vi "LVPortProcessMatlabPropertyEvents.vi"(8 "error in":errorcluster, 10 "Wait for events [ms] (0)":i32, 11 "pID":string) -> (0 "error out":errorcluster)   [LabVIEW 2017]
uses:
  Properties/LVPortControlBindingInfoType.ctl
  Properties/LVPortControlBindingDirectionEnum.ctl
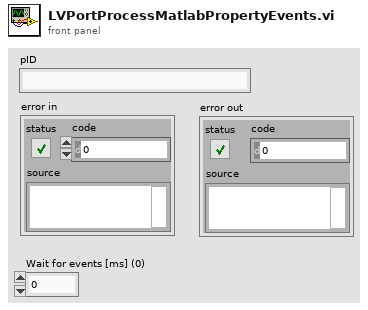
[diagram p1: front panel]
types:
  T1 = typedef "LVPortEventRegistrationDataType.ctl" = refnum<event-registration>
  T2 = typedef "LVPortControlBindingDirectionEnum.ctl" = enum16{"BiDirectional", "ToMatlab", "ToLabview"}
  T3 = typedef "LVPortControlBindingInfoType.ctl" = cluster{"Bound Control":refnum<vi>, "Name":string, "Direction":T2, "Event Register":refnum<event-registration>}
  T4 = typedef "Dictionary Object RefNum__ogtk.ctl" = refnum<k1>
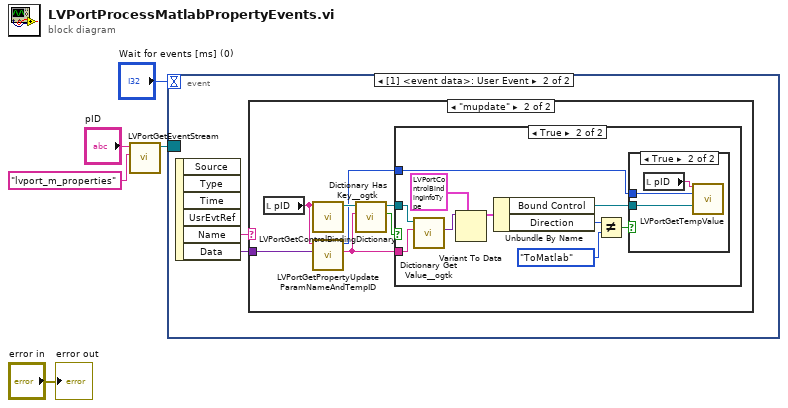
[diagram p0: block diagram]
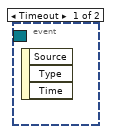
[diagram p2: hidden frame]
diagram:
  n1 = call "LVPortGetEventStream.vi"("Category"="lvport_m_properties", "ID"="pID") -> ("Event Registration Refnum out"=w3:T1)  [unwired: 6 in, 3 out]
  n2 = event shown="[1] <event data>: User Event" {
    selector: w3 -> [_ _]
    dyn-events: _ -> [_ _]
    timeout: "Wait for events [ms] (0)" -> [_ _]
    event Timeout {
      n3 = event-data() -> ()  [unwired: 1 in, 3 out]
    }
    event User Event {
      n4 = event-data() -> ("Name"=w7:string, "Data"=w6:variant)  [unwired: 1 in, 4 out]
      n5 = case shown="\"mupdate\"" w7 {
        tunnel: w6 -> [_ w14]
        frame "False", Default {
        }
        frame "mupdate" {
          n6 = local read "pID"() -> (w13:string)
          n7 = call "LVPortGetControlBindingDictionary.vi"("pID"=w13) -> ("Refnum out"=w12:T4)  [unwired: 10 in]
          n8 = call "LVPortGetPropertyUpdateParamNameAndTempID.vi"("Event Data"=w14, "pID"=w13) -> ("Param Name"=w9:string, "TempID"=w8:i32)  [unwired: 8 in]
          n9 = call <userlib>:"Dictionary Has Key__ogtk.vi"("key"=w9, "dictionary"=w12) -> ("Has Key?"=w11:bool, "dictionary out"=w10:T4)  [unwired: 7 in, 1 out]
          n10 = case shown="True" w11 {
            tunnel: w10 -> [_ w23]
            tunnel: w9 -> [_ w24]
            tunnel: w8 -> [_ w18]
            frame False {
            }
            frame True {
              n11 = call <userlib>:"Dictionary Get Value__ogtk.vi"("key"=w24, "dictionary"=w23) -> ("value"=w22:variant)  [unwired: 6 in, 3 out]
              n12 = Variant To Data(type=T3 {"Bound Control"=refnum, "Name"="", "Direction"=enum."BiDirectional", "Event Register"=refnum} ("Control Binding Info"), Variant=w22) -> (data=w20:T3)  [unwired: 1 in, 1 out]
              n13 = Unbundle By Name(w20) -> ("Bound Control"=w19:refnum<vi>, "Direction"=w17:T2)
              n14 = Not Equal?(x=w17, y=LVPortControlBindingDirectionEnum."ToMatlab") -> (x != y?=w15:bool)
              n15 = case shown="True" w15 {
                tunnel: w19 -> [_ w27]
                tunnel: w18 -> [_ w26]
                frame False {
                }
                frame True {
                  n16 = local read "pID"() -> (w25:string)
                  n17 = call "LVPortGetTempValue.vi"("pID"=w25, "Object ID"=w26, "Value Type (Or value to update)"=w27) -> ()  [unwired: 10 in, 3 out]
                }
              }
            }
          }
        }
      }
    }
  }
  "error out" <- "error in"
